vi "Enable Voltage Auto Ranging.vi"(8 "error in (no error)":errorcluster, 9 "Enable Auto Range (T: Enable)":bool=TRUE, 10 "Channel (1: 1)":i32(ring)=1 items=["1"=1, "2"=2], 11 "VISA resource name":refnum<visa-resource-name>) -> (0 "error out":errorcluster, 3 "VISA resource name out":refnum<visa-resource-name>)   [LabVIEW 2015, in "Agilent 3352X Series.lvlib"]
doc: "Enables or disables voltage auto ranging. \nWith autoranging enabled, the waveform generatorc automatically selects the optimal settings for the attenuators; \nWith autoranging disabled, the waveform generator uses the current attenuator settings and does not switch attenuator relays.\n\n<b>Note</b>:\n(1) This VI does not check the instrument status. \n(2) You can disable autoranging to eliminate momentary disruptions caused by switching of the attenuators while changing amplitude. However, the amplitude and offset accuracy and resolution (as well as waveform fidelity) may be adversely affected when reducing the amplitude below the expected range change. \n(3) You may not be able to achieve the minimum aplitude that is available with autoraging on."
uses:
  <instrlib>/Agilent 3352X Series/Agilent 3352X Series.lvlib
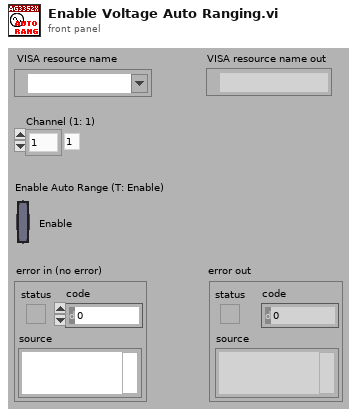
[diagram p1: front panel]
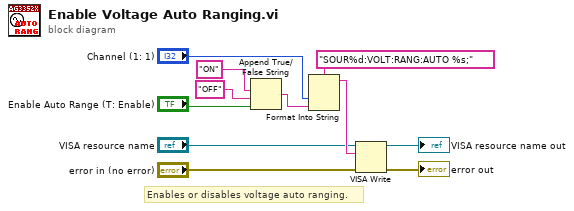
[diagram p0: block diagram]
diagram:
  # "Enables or disables voltage auto ranging."
  n1 = Append True/False String(1:"Enable Auto Range (T: Enable)", 2:"OFF", 3:"ON") -> (0:w6:string)  [unwired: 1 out]
  n2 = Format Into String(format string="SOUR%d:VOLT:RANG:AUTO %s;", "Channel (1: 1)", w6) -> (resulting string=w5:string)  [unwired: 2 in, 1 out]
  n3 = VISA Write(VISA resource name="VISA resource name", write buffer=w5, error in (no error)="error in (no error)") -> (VISA resource name out=→"VISA resource name out":refnum<visa-resource-name>, error out=→"error out":errorcluster)  [unwired: 1 out]
